vi "DAQacquire_diag.vi"(0 "LD Signal":tag="Dev3/ai0" caption="LD Channel", 1 "Samples per Channel":i32=50000 caption="LD # Samples", 5 "Reference Signal":tag="Dev3/ai2", 6 "Minimum Value":dbl=-6.0 caption="LD min Value" format="%0.2f", 9 "Error In":errorcluster, 11 "Maximum Value":dbl=-4.5 caption="LD max Value" format="%0.2f", 12 "Rate":dbl=500.0 caption="Sample Rate (Hz)" format="%0.2f") -> (3 "Reference Signal":waveform(dbl)(graph)={"t0"=timestamp(0 s since 1904-01-01), "dt"=0.002, "Y"=array[50000 elements]}, 4 "LD Signal":waveform(dbl)(graph)={"t0"=timestamp(0 s since 1904-01-01), "dt"=0.002, "Y"=array[50000 elements]}, 8 "Frequency":dbl[](array[numeric])=[5.19], 10 "Error Out":errorcluster, 13 "Measured 2f Frequency (Hz)":dbl=5.494528035395369, 14 "Peak Amplitude":dbl=0.00028966950578474833, 15 "DAQ Spectrum analyzer":cluster{"f0":dbl, "df":dbl, "magnitude":dbl[]}[](graph)=[{"f0"=0.0, "df"=0.01, "magnitude"=array[25000 elements]}, {"f0"=0.0, "df"=0.01, "magnitude"=array[25000 elements]}])   [LabVIEW 2011]
doc: "I. Description:\nThis example demonstrates how to acquire a finite amount of data (waveform) using the DAQ device's internal clock.\n\nII. Instructions for Running:\n1. Select the physical channel to correspond to where your signal is input on the DAQ device.\n2. Enter the minimum and maximum voltages.\nNote: For better accuracy try to match the input range to the expected voltage level of the measured signal.\n3. Select the number of samples to acquire.\n4. Set the rate of the acquisition\nNote: The rate should be AT LEAST twice as fast as the maximum frequency component of the signal being acquired.\n\nIII. Block Diagram Steps:\n1. Create an analog input voltage channel.\n2. Set the rate for the sample clock. Additionally, define the sample mode to be finite and set the number of samples to be acquired per channel.\n3. Call the Start VI to start the acquisition.\n4. Use the Read VI to measure multiple samples from N Channels on the device. Set a timeout so an error is returned if the samples are not returned in the specified time limit\n5. Call the Clear Task VI to clear the Task.\n6. Use the popup dialog box to display an error if any.\n \nIV. I/O Connections Overview:\nMake sure your signal input terminal matches the Physical Channel I/O Control. For further connection information, refer to your hardware reference manual."
uses:
  <vilib>/DAQmx/create/channels.llb/DAQmx Create Channel (AI-Voltage-Basic).vi
  <vilib>/measure/mascope.llb/Pulse Measurements 1 chan.vi
  <vilib>/express/express analysis/Spectral/Block/exnSpectralBlock spectral measurements RMS poly.vi
  <vilib>/express/express analysis/Spectral/Block/exnSpectralBlock spectral measurements RMS WFM.vi
  <vilib>/express/express analysis/Spectral/XNode/ExpressSpectralMeasurementsBlockNode.xnode
  <vilib>/measure/NI_MAPro.lvlib
panel:
  in  "Ref Rate (Hz)":dbl=500.0
  in  "Ref # Samples":i32=5000
  out "FFT - (RMS)":cluster{"f0":dbl, "df":dbl, "magnitude":dbl[]}={"f0"=0.0, "df"=0.01, "magnitude"=array[25000 elements]}
  # "For instructions, select Help>>Show Context Help"
  # "Channel Parameters"
  # "Timing Parameters"
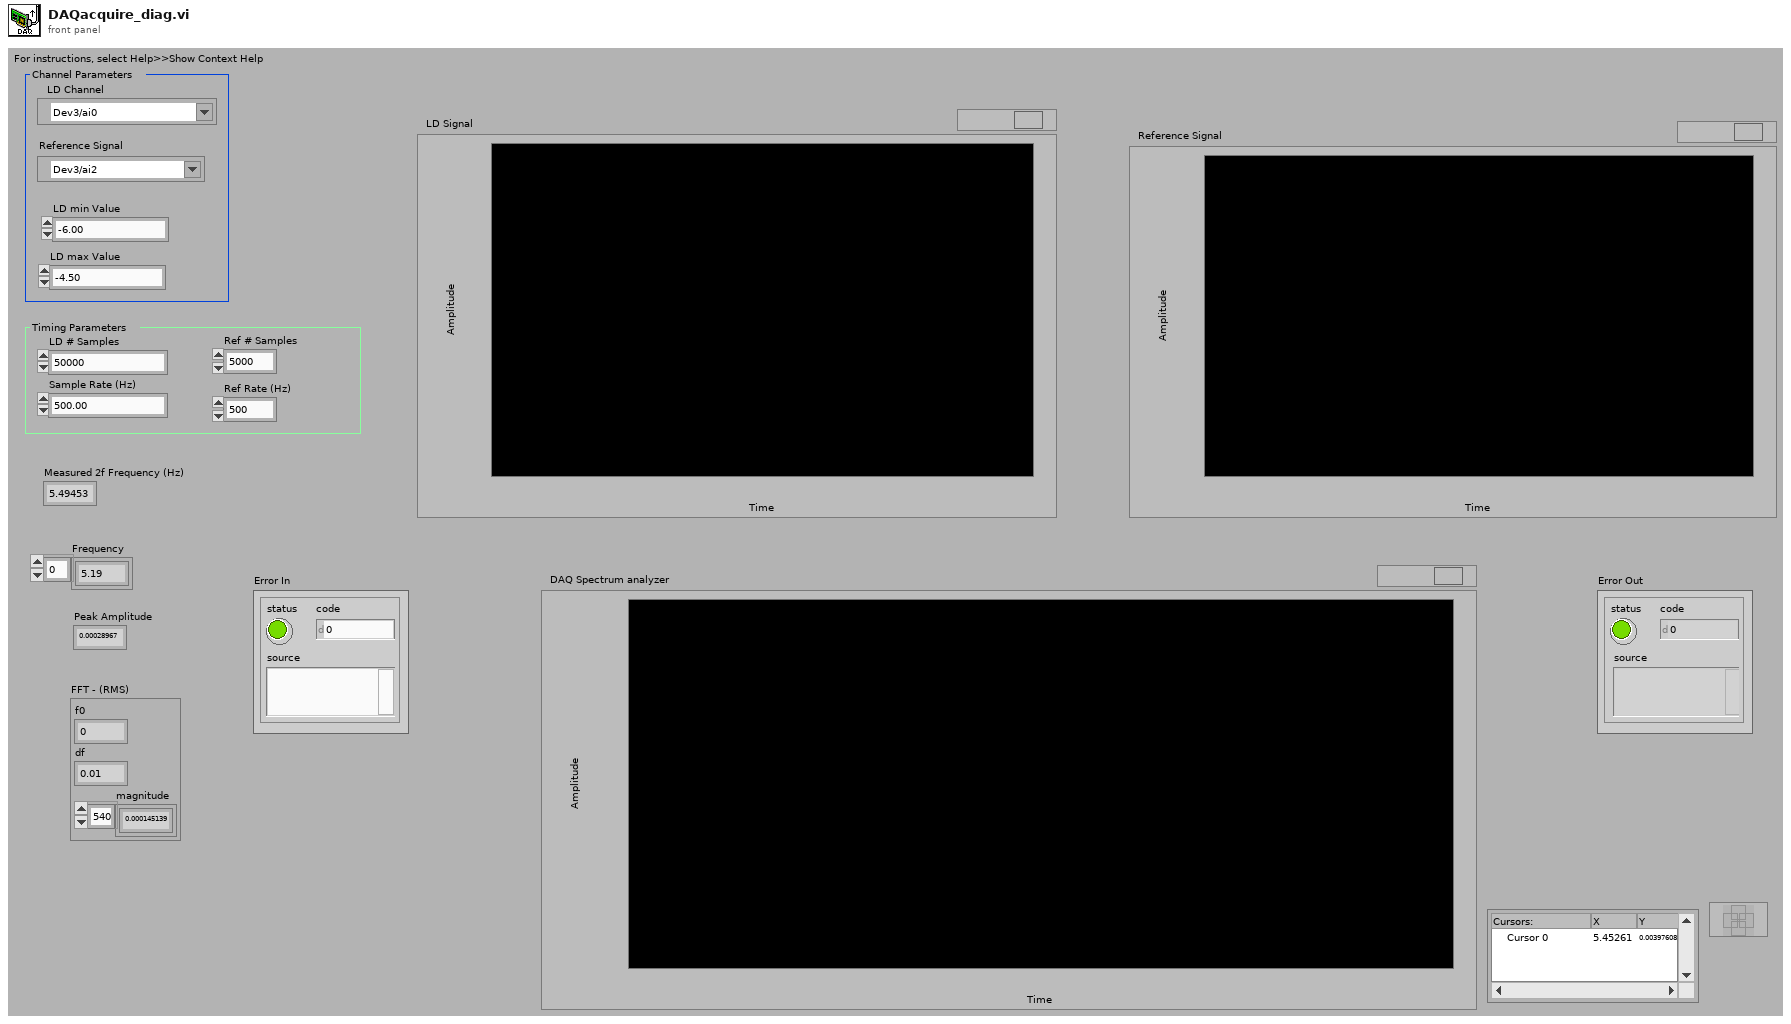
[diagram p1: front panel]
types:
  T1 = cluster{"averaging mode":u16, "weighting mode":u16, "number of averages":u32}
  T2 = cluster{"dB On (F)":bool, "unwrap phase (F)":bool, "convert to degree (F)":bool}
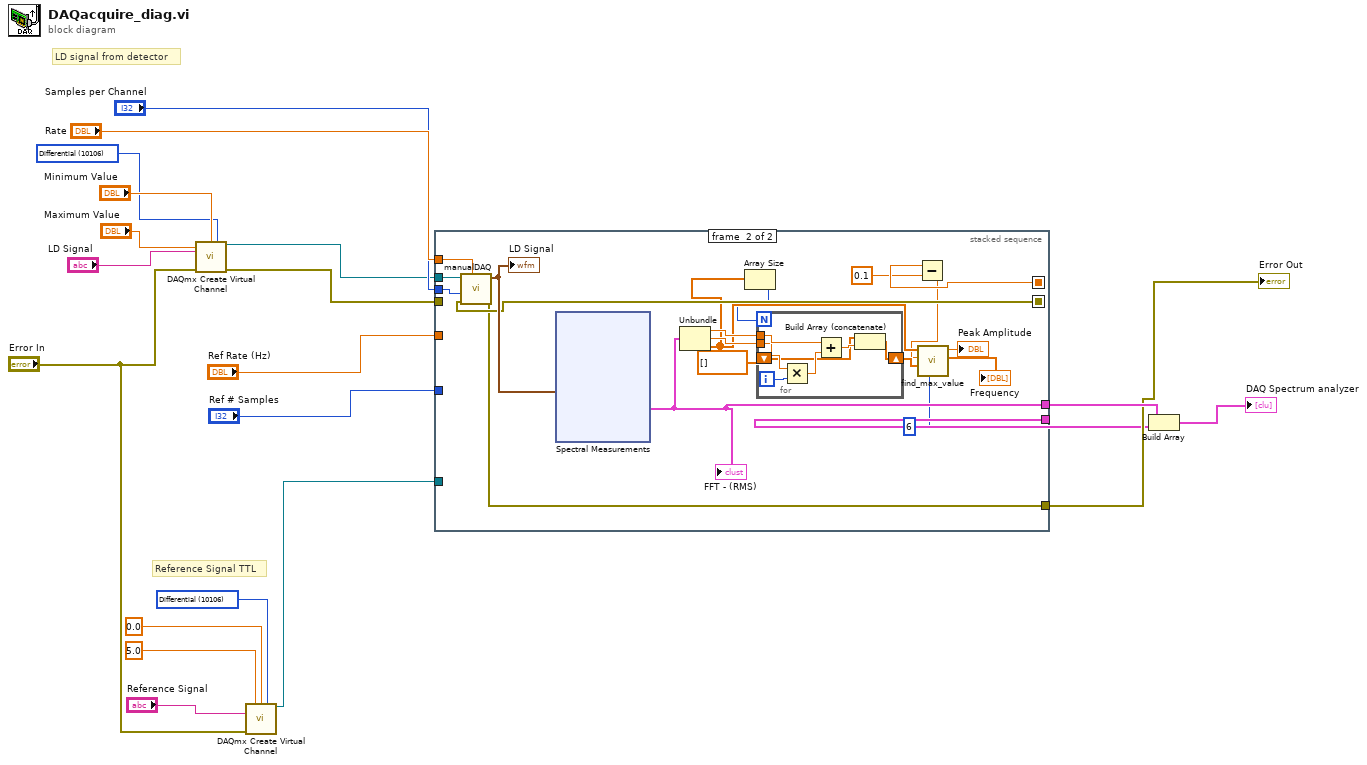
[diagram p0: block diagram]
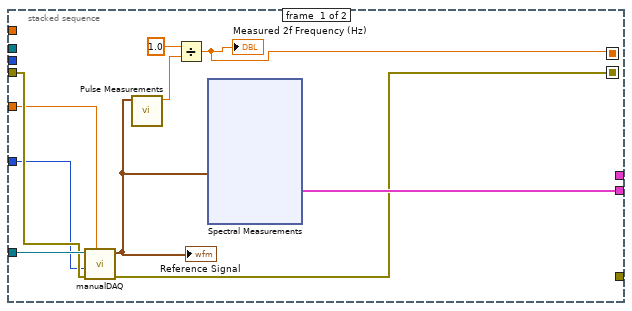
[diagram p2: hidden frame]
diagram:
  w13 = 10106 items=["default"=-1, "RSE"=10083, "NRSE"=10078, "Differential"=10106, "Pseudodifferential"=12529] ("input terminal configuration")
  w17 = 10106 items=["default"=-1, "RSE"=10083, "NRSE"=10078, "Differential"=10106, "Pseudodifferential"=12529] ("input terminal configuration")
  # "Reference Signal TTL"
  # "LD signal from detector"
  n1 = call-poly <vilib>:"DAQmx Create Virtual Channel.vi"("maximum value"="Maximum Value", "minimum value"="Minimum Value", "input terminal configuration"=w17, "physical channels"="LD Signal", "error in"="Error In") -> ("task out"=w10:refnum<k21>, "error out"=w9:errorcluster)  [unwired: 9 in]
  n2 = call-poly <vilib>:"DAQmx Create Virtual Channel.vi"("maximum value"=5.0, "minimum value"=0.0, "input terminal configuration"=w13, "physical channels"="Reference Signal", "error in"="Error In") -> ("task out"=w8:refnum<k21>)  [unwired: 9 in, 1 out]
  n3 = stacked-sequence {
    seq-local: [w24 _] -> [_ w55]
    seq-local: [w23 _] -> [_ w46]
    tunnel: "Rate" -> [_ w59]
    tunnel: "Samples per Channel" -> [_ w58]
    tunnel: w10 -> [_ w57]
    tunnel: w9 -> [w25 _]
    tunnel: w8 -> [w30 _]
    tunnel: [_ w54] -> w4
    tunnel: [_ w53] -> w7
    tunnel: [w29 _] -> w3
    tunnel: "Ref Rate (Hz)" -> [w22 _]
    tunnel: "Ref # Samples" -> [w21 _]
    frame #0 {
      n4 = call "manualDAQ.vi"("Rate"=w22, "error in (no error)"=w25, "Samples per Channel"=w21, "Refnum in"=w30) -> ("error out"=w24:errorcluster, "output waveform"=w28:waveform(dbl))  [unwired: 6 in]
      "Reference Signal" <- w28
      n5 = call-poly <vilib>:"Pulse Measurements.vi"("signal in"=w28) -> ("period"=w27:dbl)  [unwired: 6 in, 4 out]
      n6 = Divide(x=1.0, y=w27) -> (x/y=w23:dbl)
      "Measured 2f Frequency (Hz)" <- w23
      n7 = xnode "Spectral Measurements"("Signals"=w28) -> ("FFT - (RMS)"=w29:cluster{"f0":dbl, "df":dbl, "magnitude":dbl[]})  [unwired: 1 in, 2 out]
    }
    frame #1 {
      n8 = call "manualDAQ.vi"("Rate"=w59, "error in (no error)"=w55, "Samples per Channel"=w58, "Refnum in"=w57) -> ("error out"=w54:errorcluster, "output waveform"=w56:waveform(dbl))  [unwired: 6 in]
      "LD Signal" <- w56
      n9 = xnode "Spectral Measurements"("Signals"=w56) -> ("FFT - (RMS)"=w53:cluster{"f0":dbl, "df":dbl, "magnitude":dbl[]})  [unwired: 1 in, 2 out]
      "FFT - (RMS)" <- w53
      n10 = Unbundle(w53) -> ("f0"=w52:dbl, "df"=w51:dbl, "magnitude"=w50:dbl[])
      n11 = Array Size(array=w50) -> (size(s)=w49:i32)
      n12 = for {
        N: w49 -> [_]
        tunnel: w52 -> [w66]
        tunnel: w51 -> [w63]
        shift-right: [w61] -> w47
        shift-left: dbl[] [] -> [w60]
        i -> [w65]
        n13 = Multiply(x=w63, y=w65) -> (x*y=w64:dbl)
        n14 = Add(x=w66, y=w64) -> (x+y=w62:dbl)
        n15 = Build Array (concatenate)(w60, w62) -> (w61:dbl[])
      }
      n16 = Subtract(x=w46, y=0.1) -> (x-y=w44:dbl)
      n17 = call "find_max_value.vi"("length"=6, "Frequency array"=w47, "Lower Freq"=w44, "Amplitude Array"=w50) -> ("Frequency"=→"Frequency":dbl[], "Peak Amplitude"=→"Peak Amplitude":dbl)  [unwired: 6 in]
    }
  }
  "Error Out" <- w4
  n18 = Build Array(w7, w3) -> (→"DAQ Spectrum analyzer":cluster{"f0":dbl, "df":dbl, "magnitude":dbl[]}[])
